vi "HealthAndStatusRequest.vi"(1 "HealthAndStatusSize":u32) -> ()   [LabVIEW 2016]
uses:
  <vilib>/rvi/Emulation/niFpgaEmulationIsFPGAContextNoSignature.vi
  <vilib>/rvi/Emulation/niFpgaSctlEmulationGetInTimedLoop.vi
  <vilib>/rvi/errors/niFpgaSetErrorForExecOnDevCompSimple.vi
  <vilib>/rvi/eio/common/nirviEmuReportErrorAndStop.vi
  <vilib>/rvi/DataTransferAndStorage/Container/Common/niFpgaContainerGetUniqueNameForEmu.vi
  <vilib>/rvi/FIFO/Fifo_Resource/nirvififoEmulationSetSize.vi
  <vilib>/rvi/FIFO/Fifo_Resource/nirviFifoEmulationQueueMgr.vi
  <instcachedir>/0/nirviFifoEmulationQueueMgr_E5CAEC123FF24DC58D834DCA3CDAA9B5.lvgen/nirviFifoEmulationQueueMgr_E5CAEC123FF24DC58D834DCA3CDAA9B5_007.vi
  <vilib>/rvi/FIFO/Fifo_Resource/nirvififoEmulationDetermineInputValidOut.vi
  <vilib>/rvi/FIFO/Fifo_Resource/nirvififoEmulationCreateLock.vi
  <vilib>/rvi/Emulation/niFpgaProcessEmulError.vi
  <vilib>/rvi/FIFO/Fifo_Resource/nirvififoEmulationObtainLock.vi
  <vilib>/rvi/FIFO/Fifo_Resource/nirvififoEmulationReleaseLock.vi
  <vilib>/rvi/occurrence/nirviWaitOnOccurrenceBase.vi
  <vilib>/rvi/errors/nirviReportUnexpectedCaseInternalError.vi
  <vilib>/rvi/errors/nirviReportUnexpectedCaseInternalError (U32).vi
  <vilib>/rvi/DataTransferAndStorage/Container/Common/niFpgaContainerExecOnDevCompGetState.vi
  <vilib>/Utility/error.llb/Clear Errors.vi
  <vilib>/rvi/interface/RandomDataEmulation/niFpgaRandomDataHandleErrors.vi
  <vilib>/rvi/Emulation/niFpgaGetClockAttributes.vi
  <vilib>/rvi/Emulation/niFpgaEmulationReportErrorSimple.vi
  <vilib>/rvi/Emulation/niFpgaCriticalErrorInLSC.vi
  <vilib>/rvi/DataTransferAndStorage/Container/XNode/niFpgaContainer.xnode
  <vilib>/rvi/FIFO/Fifo_Resource/nirvififoEmulationWrite.vi
  <vilib>/rvi/FIFO/Fifo_Resource/niFpgaFifoEmulationRefIn.vi
  <vilib>/rvi/FIFO/Fifo_Resource/nirvififoEmulationGetNumberOfElementsToRead.vi
  <vilib>/rvi/FIFO/Fifo_Resource/nirvififoEmulationRead.vi
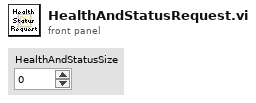
[diagram p1: front panel]
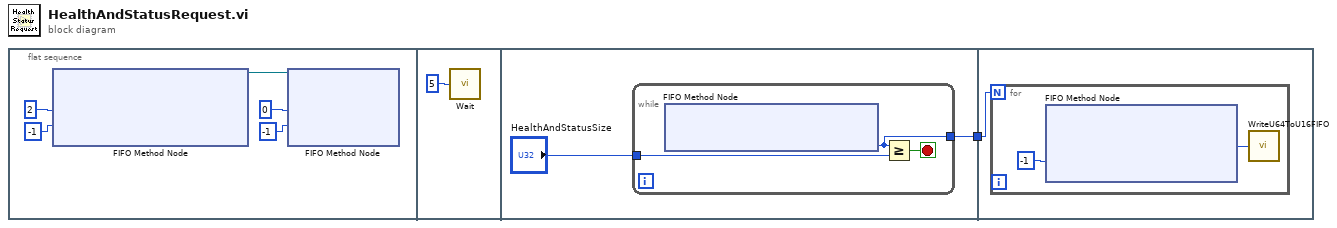
[diagram p0: block diagram]
diagram:
  n1 = flat-sequence {
    tunnel: [w9] -> w1
    tunnel: w1 -> [w13]
    frame #0 {
      n2 = xnode ("FIFO Method Node")("Element"=u64 2, "Timeout"=-1) -> ("FIFO Out"=w6:refnum<k21>)  [unwired: 1 in, 1 out]
      n3 = xnode ("FIFO Method Node")("Element"=u64 0, "Timeout"=-1, "FIFO In"=w6) -> ()  [unwired: 2 out]
    }
    frame #1 {
      n4 = call "Wait"("Count(uSec)"=u32 5) -> ()  [unwired: 1 out]
    }
    frame #2 {
      n5 = while {
        tunnel: [w11] -> w9
        tunnel: "HealthAndStatusSize" -> [w10]
        stop <- w12 stop-if-true
        n6 = xnode ("FIFO Method Node")() -> ("Number of Elements to Read"=w11:u32)  [unwired: 1 in, 1 out]
        n7 = Greater Or Equal?(x=w11, y=w10) -> (x >= y?=w12:bool)
      }
    }
    frame #3 {
      n8 = for {
        N: w13 -> [_]
        n9 = xnode ("FIFO Method Node")("Timeout"=-1) -> ("Element"=w14:u64)  [unwired: 1 in, 2 out]
        n10 = call "WriteU64ToU16FIFO.vi"("U64"=w14) -> ()  [unwired: 1 in]
      }
    }
  }
